vi "ReadSimpleBatteryState.vi"() -> (0 "measurement":dbl format="%0.2f", 1 "BatteryHealth":T1)   [LabVIEW 2021]
uses:
  Enums/BatteryHealth_Enum.ctl
  <vilib>/DAQmx/read.llb/DAQmx Read (Analog DBL 1Chan 1Samp).vi
  <vilib>/DAQmx/miscellaneous.llb/DAQmx Fill In Error Info.vi
panel:
  out "error out":errorcluster
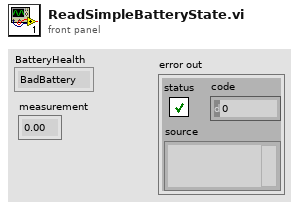
[diagram p1: front panel]
types:
  T1 = typedef "BatteryHealth_Enum.ctl" = enum16{"BadBattery", "GoodBattery"}
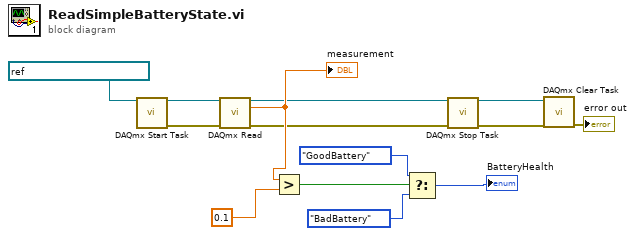
[diagram p0: block diagram]
diagram:
  n1 = call <vilib>:"DAQmx Start Task.vi"("task/channels in"=refnum<k21> "UnsignedVoltageTask") -> ("task out"=w9:refnum<k21>, "error out"=w8:errorcluster)  [unwired: 13 in]
  n2 = call-poly <vilib>:"DAQmx Read.vi"("task/channels in"=w9, "error in"=w8) -> ("task out"=w6:refnum<k21>, "data"=w7:dbl, "error out"=w5:errorcluster)  [unwired: 11 in]
  "measurement" <- w7
  n3 = Greater?(x=w7, y=0.1) -> (0:w11:bool)
  n4 = Select(t=BatteryHealth_Enum."GoodBattery" ("BatteryState 2"), s=w11, f=BatteryHealth_Enum."BadBattery" ("BatteryState 2")) -> (s? t:f=→"BatteryHealth":T1)
  n5 = call <vilib>:"DAQmx Stop Task.vi"("task/channels in"=w6, "error in"=w5) -> ("task out"=w4:refnum<k21>, "error out"=w3:errorcluster)  [unwired: 12 in]
  n6 = call <vilib>:"DAQmx Clear Task.vi"("task in"=w4, "error in"=w3) -> ("error out"=→"error out":errorcluster)  [unwired: 13 in]
